vi "InitializeLineDigital.vi"(2 "Store Data":bool, 3 "Image Settings":T1={"Start Position (µm)"={"x"=0.0, "y"=0.0, "z"=0.0}, "End Position (µm)"={"x"=10.0, "y"=10.0, "z"=0.0}, "Image Resolution (nm/pixel)"={"x"=50.0, "y"=50.0, "z"=100.0}, "Image Size (µm)"={"x"=10.0, "y"=10.0, "z"=0.0}, "Image Size (pixel)"={"x"=50, "y"=50, "z"=0}, "Time Resolution\n(ms/pixel)"=7.0, "1st Axis"=0, "2nd Axis"=1, "Retrace"=FALSE, "Estimated Time"=""} {"2nd Axis" items=["x", "y", "z"]; "1st Axis" items=["x", "y", "z"]; "Time Resolution\n(ms/pixel)" format="%.2f"; "Image Resolution (nm/pixel)"."z" format="%.2f"; "Image Resolution (nm/pixel)"."y" format="%.2f"; "Image Resolution (nm/pixel)"."x" format="%.2f"; "Image Size (µm)"."z" format="%.2f"; "Image Size (µm)"."y" format="%.2f"; "Image Size (µm)"."x" format="%.2f"; "End Position (µm)"."z" format="%.2f"; "End Position (µm)"."y" format="%.2f"; "End Position (µm)"."x" format="%.2f"; "Start Position (µm)"."z" format="%.2f"; "Start Position (µm)"."y" format="%.2f"; "Start Position (µm)"."x" format="%.2f"}, 4 "error in (no error)":errorcluster, 5 "Destination:":path) -> (0 "error out":errorcluster, 1 "Busy":bool)   [LabVIEW 2009]
uses:
  ImageSettings.ctt
panel:
  out "Velocity":dbl[](array[numeric]) format="%.6f"
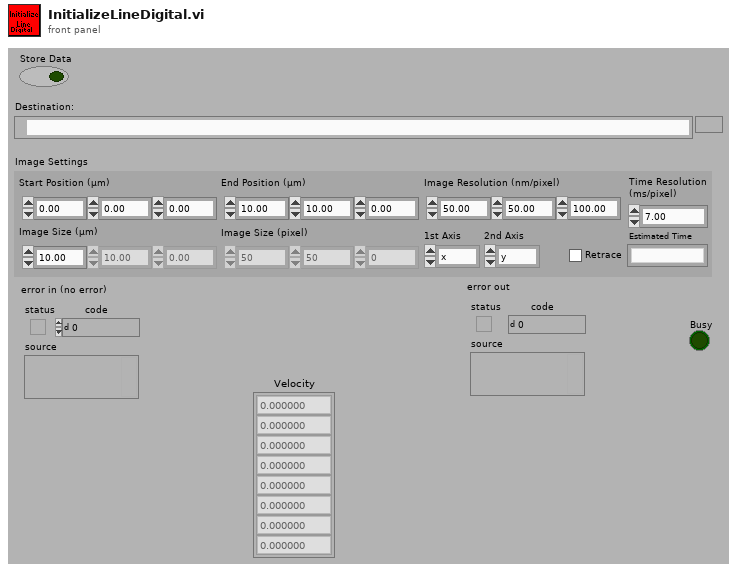
[diagram p1: front panel]
types:
  T1 = typedef "ImageSettings.ctt" = cluster{"Start Position (µm)":cluster{"x":dbl, "y":dbl, "z":dbl}, "End Position (µm)":cluster{"x":dbl, "y":dbl, "z":dbl}, "Image Resolution (nm/pixel)":cluster{"x":dbl, "y":dbl, "z":dbl}, "Image Size (µm)":cluster{"x":dbl, "y":dbl, "z":dbl}, "Image Size (pixel)":cluster{"x":u32, "y":u32, "z":u32}, "Time Resolution\n(ms/pixel)":dbl, "1st Axis":u16, "2nd Axis":u16, "Retrace":bool, "Estimated Time":string}
  T2 = typedef "LineScanStatus.ctt" = cluster{"in line":bool, "line status":cluster{"count":u32, "current":cluster{"x":u32, "y":u32, "z":u32}}, "plane status":cluster{"count":u32, "current":cluster{"x":u32, "y":u32, "z":u32}}, "new line step":cluster{"x":dbl, "y":dbl, "z":dbl}, "new plane step":cluster{"x":dbl, "y":dbl, "z":dbl}}
  T3 = cluster{"Velocity[0]":dbl, "Velocity[1]":dbl, "Velocity[2]":dbl, "Velocity[3]":dbl, "Velocity[4]":dbl, "Velocity[5]":dbl, "Velocity[6]":dbl, "Velocity[7]":dbl, "Velocity[8]":dbl}
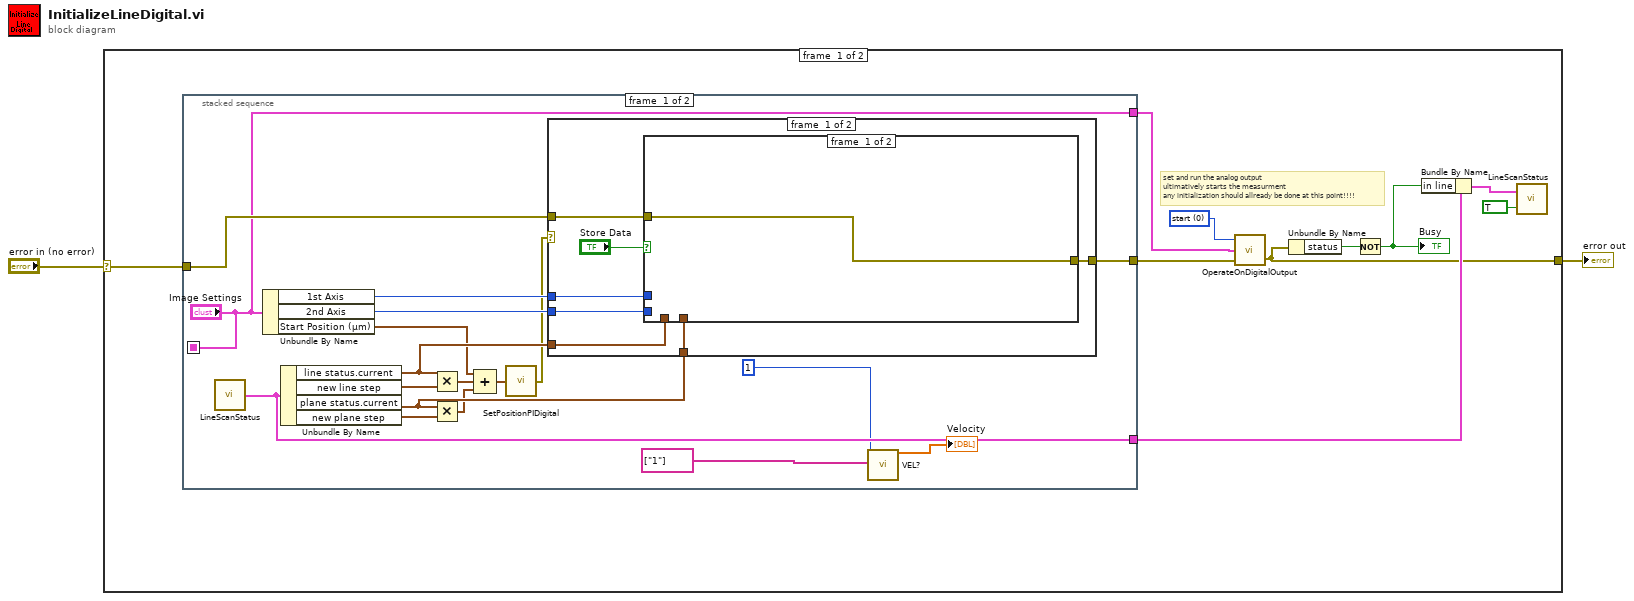
[diagram p0: block diagram]
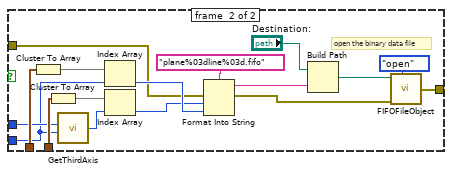
[diagram p2: hidden frame]
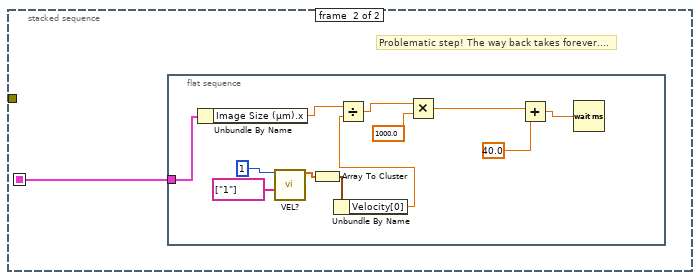
[diagram p4: hidden frame]
diagram:
  n1 = case shown="No Error" "error in (no error)" {
    selector: "error in (no error)" -> [w8 w70]
    tunnel: [w6 w70] -> w2
    frame #0 {
      w4 = u16 0 items=["start", "state", "abort"] ("operation")
      # "set and run the analog output\nultimatively starts the measurment\nany initialization should allready be done at this point!!!!"
      n2 = stacked-sequence {
        seq-local: ["Image Settings" _] -> [_ w57]
        tunnel: [w26 _] -> w10
        tunnel: w8 -> [w25 _]
        tunnel: [w20 _] -> w5
        tunnel: ["Image Settings" _] -> w3
        frame #0 {
          n3 = call "LineScanStatus.vi"() -> ("Linescan Status (output)"=w26:T2)  [unwired: 2 in]
          n4 = Unbundle By Name("Image Settings") -> ("1st Axis"=w24:u16, "2nd Axis"=w23:u16, "Start Position (µm)"=w17:cluster{"x":dbl, "y":dbl, "z":dbl})
          n5 = Unbundle By Name(w26) -> ("line status.current"=w28:cluster{"x":u32, "y":u32, "z":u32}, "new line step"=w30:cluster{"x":dbl, "y":dbl, "z":dbl}, "plane status.current"=w27:cluster{"x":u32, "y":u32, "z":u32}, "new plane step"=w29:cluster{"x":dbl, "y":dbl, "z":dbl})
          n6 = Multiply(x=w28, y=w30) -> (x*y=w22:cluster{"x":dbl, "y":dbl, "z":dbl})
          n7 = Multiply(x=w27, y=w29) -> (x*y=w21:cluster{"x":dbl, "y":dbl, "z":dbl})
          n8 = Compound Arithmetic op=ADD(w17, w22, w21) -> (w19:cluster{"x":dbl, "y":dbl, "z":dbl})
          n9 = call "SetPositionPIDigital.vi"("Current Position (µm) 2"=w19) -> ("error out 2"=w18:errorcluster)
          n10 = case shown="No Error" w18 {
            selector: w18 -> [_ w56]
            tunnel: w28 -> [w37 _]
            tunnel: w27 -> [w36 _]
            tunnel: w25 -> [w35 _]
            tunnel: w24 -> [w34 _]
            tunnel: w23 -> [w33 _]
            tunnel: [w32 w56] -> w20
            frame #0 {
              n11 = case shown="False" "Store Data" {
                tunnel: w37 -> [_ w55]
                tunnel: w36 -> [_ w54]
                tunnel: w35 -> [w38 w48]
                tunnel: w34 -> [_ w47]
                tunnel: w33 -> [_ w46]
                tunnel: [w38 w39] -> w32
                frame #0 {
                }
                frame #1 {
                  # "open the binary data file"
                  n12 = Cluster To Array(cluster=w55) -> (array=w51:u32[])
                  n13 = Cluster To Array(cluster=w54) -> (array=w50:u32[])
                  n14 = call "GetThirdAxis.vi"("1st Axis"=w46, "2nd Axis"=w47) -> ("3rd Axis"=w49:i32)  [unwired: 2 in]
                  n15 = Index Array(array=w51, index=w46) -> (element=w53:u32)
                  n16 = Index Array(array=w50, index=w49) -> (element=w52:u32)
                  n17 = Format Into String(format string="plane%03dline%03d.fifo", error in=w48, w52, w53) -> (resulting string=w44:string, error out=w40:errorcluster)  [unwired: 1 in]
                  n18 = Build Path(base path="Destination:", name or relative path=w44) -> (appended path=w45:path)
                  n19 = call "FIFOFileObject.vi"("function (open:0)"=enum16{"open", "write", "close"}."open", "error in (no error)"=w40, "Destination:"=w45) -> ("error out"=w39:errorcluster)  [unwired: 3 in]
                }
              }
            }
            frame #1 {
            }
          }
          n20 = call "VEL?.vi"("System no."=1, "Axes to query"=string[] ["1"] ("Axes to move")) -> ("Velocity"=→"Velocity":dbl[])  [unwired: 16 in, 1 out]
        }
        frame #1 {
          # "Problematic step! The way back takes forever...."
          n21 = flat-sequence {
            tunnel: w57 -> [w59]
            frame #0 {
              n22 = Unbundle By Name(w59) -> ("Image Size (µm).x"=w58:dbl)
              n23 = call "VEL?.vi"("System no."=1, "Axes to query"=string[] ["1"]) -> ("Velocity"=w64:dbl[])  [unwired: 16 in, 1 out]
              n24 = Array To Cluster(array=w64) -> (cluster=w65:T3)
              n25 = Unbundle By Name(w65) -> ("Velocity[0]"=w63:dbl)
              n26 = Divide(x=w58, y=w63) -> (x/y=w62:dbl)
              n27 = Multiply(x=w62, y=1000.0) -> (x*y=w60:dbl)
              n28 = Add(x=w60, y=40.0) -> (x+y=w66:dbl)
              n29 = Wait (ms)(milliseconds to wait=w66) -> ()  [unwired: 1 out]
            }
          }
        }
      }
      n30 = call "OperateOnDigitalOutput.vi"("error in (no error)"=w5, "Image Settings"=w3, "operation"=w4) -> ("error out"=w6:errorcluster)  [unwired: 1 in]
      n31 = Unbundle By Name(w6) -> ("status"=w7:bool)
      n32 = Not(x=w7) -> (.not. x?=w9:bool)
      "Busy" <- w9
      n33 = Bundle By Name(cluster=w10, "in line"=w9) -> (w11:T2)
      n34 = call "LineScanStatus.vi"("Get/Set"=TRUE, "Linescan Status (input)"=w11) -> ()  [unwired: 1 out]
    }
    frame #1 {
    }
  }
  "error out" <- w2
